vi "Get Transfer Mode.vi"(1 "GOLPI ref.":T2={"pipe handle"={"lv_proc.dll file path"=path "", "process instance handle"=[], "debug mode"=FALSE, "debug data"=[]}, "fast read timeout [ms]"=500, "fast read settle time [ms]"=10, "fast read to multiple [ms]"=1, "max elements per input line"=100, "slow read timeout [ms]"=5000, "stdin double format specifier"="%_16e", "max elements per stdout output column"=100, "console mode bitstream"=FALSE, "bitstream first read timeout [ms]"=1000, "bitstream read timeout [ms]"=50, "struct transfer possible"=FALSE, "matlab mode"=FALSE, "var pipe write timeout [ms]"=5000, "variable pipe mode"=FALSE, "variable pipe buffer size [Bytes]"=10000000, "variable pipe block size [Bytes]"=1000000} {"variable pipe block size [Bytes]" format="%.0p"; "variable pipe buffer size [Bytes]" format="%.0p"}, 2 "use temporary file? (F)":bool) -> (0 "mode":T1)   [LabVIEW 2020, in "GOLPI library.lvlib"]
doc: "Get configured variable transfer mode from GOLPI reference."
uses:
  GOLPI library.lvlib
  Public/GOLPI reference Type Def.ctl
  LV Process source distribution/Pipe Handle.ctl
  Type Definitions/Transfer Mode.ctl
  LV Process source distribution/LV Process library.lvlib
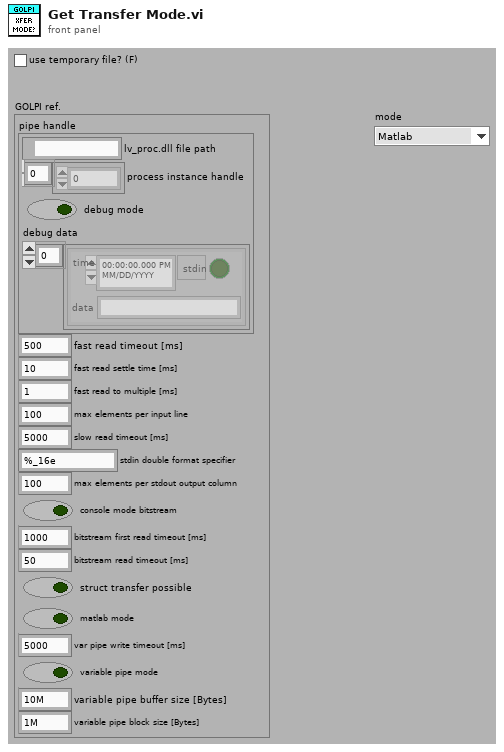
[diagram p1: front panel]
types:
  T1 = typedef "GOLPI library.lvlib/Transfer Mode.ctl" = enum16{"Matlab", "stdio", "temp file", "bitstream", "pipe"}
  T2 = typedef "GOLPI library.lvlib/GOLPI reference Type Def.ctl" = cluster{"pipe handle":T3, "fast read timeout [ms]":u32, "fast read settle time [ms]":u32, "fast read to multiple [ms]":u32, "max elements per input line":u32, "slow read timeout [ms]":u32, "stdin double format specifier":string, "max elements per stdout output column":u32, "console mode bitstream":bool, "bitstream first read timeout [ms]":u32, "bitstream read timeout [ms]":u32, "struct transfer possible":bool, "matlab mode":bool, "var pipe write timeout [ms]":u32, "variable pipe mode":bool, "variable pipe buffer size [Bytes]":u32, "variable pipe block size [Bytes]":u32}
  T3 = typedef "LV Process library.lvlib/Pipe Handle.ctl" = cluster{"lv_proc.dll file path":path, "process instance handle":u32[], "debug mode":bool, "debug data":cluster{"time":timestamp, "stdin":bool, "data":string}[]}
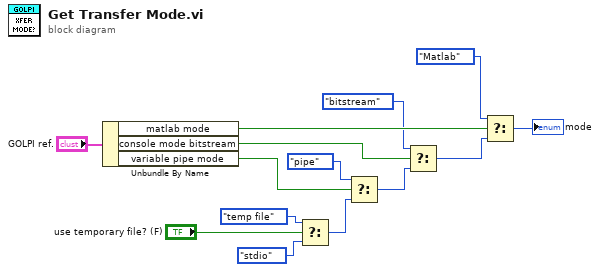
[diagram p0: block diagram]
diagram:
  n1 = Unbundle By Name("GOLPI ref.") -> ("matlab mode"=w13:bool, "console mode bitstream"=w11:bool, "variable pipe mode"=w7:bool)
  n2 = Select(t=Transfer_Mode."temp file" ("f"), s="use temporary file? (F)", f=Transfer_Mode."stdio") -> (s? t:f=w5:T1)
  n3 = Select(t=Transfer_Mode."pipe" ("mode"), s=w7, f=w5) -> (s? t:f=w8:T1)
  n4 = Select(t=Transfer_Mode."bitstream" ("mode"), s=w11, f=w8) -> (s? t:f=w10:T1)
  n5 = Select(t=Transfer_Mode."Matlab" ("mode"), s=w13, f=w10) -> (s? t:f=→"mode":T1)
